vi "Modbus_Escribe.vi"(9 "register values":u16[](array[numeric])=[0]) -> ()   [LabVIEW 2019, in "Class 2.lvclass"]
uses:
  Class 2.lvclass
  <vilib>/NI/Modbus Library/API/Wrapper/Create TCP Master.vi
  <vilib>/NI/Modbus Library/API/Master/Modbus Master.lvclass
  <vilib>/NI/Modbus Library/API/Wrapper/API Main.lvlib
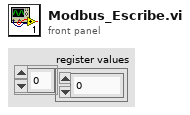
[diagram p1: front panel]
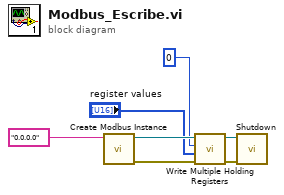
[diagram p0: block diagram]
diagram:
  n1 = call-poly <vilib>:"Create Modbus Instance.vi"("address"="0.0.0.0") -> ("error out"=w5:errorcluster, "TCP master instance"=w6:refnum<class "Modbus Master.lvclass">)  [unwired: 9 in]
  n2 = call-dynamic "Write Multiple Holding Registers.vi"("error in"=w5, "registers to write"="register values", "starting address"=u16 0, "Modbus master in"=w6) -> ("error out"=w4:errorcluster, "Modbus master out"=w3:refnum<class "Modbus Master.lvclass">)  [unwired: 6 in]
  n3 = call-dynamic "Shutdown.vi"("error in"=w4, "Modbus master in"=w3) -> ()  [unwired: 9 in, 1 out]
